vi "HFRR ADV v02.vi"() -> ()   [LabVIEW 2025] (continued)
          tunnel: [FALSE ("RUN") TRUE ("RUN")] -> w2596
          tunnel: [_ 2] -> w2590
          frame False {
          }
          frame True {
          }
        }
        n2286 = case shown="True" w2595 {
          tunnel: [FALSE ("RUN") TRUE ("RUN")] -> w2594
          tunnel: [_ 3] -> w2589
          frame False {
          }
          frame True {
          }
        }
        n2287 = case shown="\"Acquire\"" w2575 {
          tunnel: w2577 -> [_ w2808]
          frame Default {
            w2807 = 0.0 ("output")
            n2288 = local write "PID-out"(w2807) -> ()
            n2289 = local write "Frequency ( Hz )"(w2807) -> ()
          }
          frame "Acquire" {
            n2290 = stacked-sequence {
              frame #0 {
                n2291 = local read "Auto Start Test"() -> (w2810:bool)
                n2292 = case shown="True" w2810 {
                  tunnel: "RUN" -> [w2831 w2834]
                  tunnel: [w2831 w2833] -> w2811
                  frame False {
                  }
                  frame True {
                    n2293 = local read "Auto Start Temp"() -> (w2832:bool)
                    n2294 = Or(x=w2834, y=w2832) -> (x .or. y?=w2833:bool)
                  }
                }
                n2295 = local read "clk"() -> (w2830:dbl)
                n2296 = local read "Save"() -> (w2826:bool)
                n2297 = Equal?(x=w2830, y=0.0) -> (x = y?=w2827:bool)
                n2298 = And(x=w2827, y=w2826) -> (x .and. y?=w2828:bool)
                n2299 = Not(x="Engage") -> (.not. x?=w2817:bool)
                n2300 = case shown="True" w2811 {
                  tunnel: [0.0 w2851] -> w2813
                  frame False {
                    (unwired) TRUE ("Visible")
                    n2301 = local read "Auto Start Test"() -> (w2838:bool)
                    n2302 = local write "Start Time"(TRUE ("Start Time")) -> ()
                    n2303 = property on="Stroke 2" class="DigNum (strict)"("Visible"=FALSE) -> ()  [unwired: 2 in, 2 out]
                    n2304 = case shown="False" w2838 {
                      frame False {
                        n2305 = property on="Heater Button" class="Bool (strict)"("DisabledEnum"=T13."Enabled" ("Disabled")) -> ()  [unwired: 2 in, 2 out]
                        n2306 = property on="Humidity" class="Bool (strict)"("DisabledEnum"=T13."Enabled" ("Disabled")) -> ()  [unwired: 2 in, 2 out]
                      }
                      frame True {
                      }
                    }
                    n2307 = case shown="False" "TestCompFlg" {
                      frame False {
                        n2308 = local read "StartFlg"() -> (w2846:bool)
                        n2309 = case shown="True" w2846 {
                          frame False {
                          }
                          frame True {
                            n2310 = flat-sequence {
                              frame #0 {
                                n2311 = local read "EVENT LOG"() -> (w2848:string)
                                n2312 = call "Event Log.vi"("Content"="Test was interrupted", "EVENT LOG"=w2848) -> ("EVENT LOG"=w2849:string)  [unwired: 8 in, 1 out]
                                n2313 = local write "EVENT LOG"(w2849) -> ()
                              }
                              frame #1 {
                                w2850 = FALSE ("StartFlg")
                                n2314 = local write "Heater Button"(w2850) -> ()
                                n2315 = local write "StartFlg"(w2850) -> ()
                                n2316 = local write "Humidity"(w2850) -> ()
                              }
                            }
                          }
                        }
                      }
                      frame True {
                      }
                    }
                    n2317 = local write "String 14"("Test will autostart once parameters reach the set value." ("String 14")) -> ()
                  }
                  frame True {
                    (unwired) FALSE ("Visible")
                    n2318 = property on="Stroke 2" class="DigNum (strict)"("Visible"=TRUE) -> ()  [unwired: 2 in, 2 out]
                    n2319 = property on="STOP 2" class="Bool (strict)"("Disabled"=u8 2) -> ()  [unwired: 2 in, 2 out]
                    n2320 = local write "String 14"(" Running....." ("String 14")) -> ()
                    n2321 = property on="Heater Button" class="Bool (strict)"("DisabledEnum"=T13."Disabled and Grayed Out" ("Disabled")) -> ()  [unwired: 2 in, 2 out]
                    n2322 = property on="Humidity" class="Bool (strict)"("DisabledEnum"=T13."Disabled and Grayed Out" ("Disabled")) -> ()  [unwired: 2 in, 2 out]
                    n2323 = case shown="True" "Start Time" {
                      selector: "Start Time" -> [_ w2864]
                      frame False {
                      }
                      frame True {
                        n2324 = Not(x=w2864) -> (.not. x?=w2863:bool)
                        n2325 = local write "Start Time"(w2863) -> ()
                        n2326 = local read "EVENT LOG"() -> (w2865:string)
                        n2327 = call "Event Log.vi"("Content"="Test in progress", "EVENT LOG"=w2865) -> ("EVENT LOG"=w2867:string)  [unwired: 8 in, 1 out]
                        n2328 = local write "EVENT LOG"(w2867) -> ()
                      }
                    }
                    n2329 = local read "Set Hz"() -> (w2861:dbl)
                    n2330 = call <vilib>:"Uniform White Noise Waveform.vi"() -> ("signal out"=w2860:waveform(dbl))  [unwired: 10 in, 1 out]
                    n2331 = Add(x=w2861, y=w2860) -> (x+y=w2859:waveform(dbl))
                    n2332 = Multiply(x=w2859, y=ext 0.1) -> (x*y=w2851:waveform(ext))
                    "StartFlg" <- TRUE ("StartFlg")
                  }
                }
                n2333 = case shown="True" w2828 {
                  frame False {
                  }
                  frame True {
                    n2334 = local write "clk"(10.0 ("clk")) -> ()
                    n2335 = Get Date/Time In Seconds() -> (seconds since 1Jan1904=w2870:timestamp)
                    n2336 = To Double Precision Float(number=w2870) -> (double precision float=w2868:dbl)
                    n2337 = local write "acq timer"(w2868) -> ()
                    n2338 = local write "act save time"(w2868) -> ()
                  }
                }
                n2339 = call "Elapsed Time"("Time Target (s)"="Countdown", "Reset"=w2817) -> ("Elapsed Time (s)"=w2822:dbl, "Time has Elapsed"=w2820:bool)  [unwired: 10 in, 6 out]
                "Countdown 2" <- w2822
                n2340 = Subtract(x=w2822, y=2.0) -> (x-y=w2825:dbl)
                n2341 = Less?(x=w2825, y="Countdown") -> (x < y?=w2823:bool)
                n2342 = And(x=w2823, y=w2820) -> (x .and. y?=w2819:bool)
                n2343 = case shown="True" w2819 {
                  frame False {
                  }
                  frame True {
                    (unwired) dbl[] [] ("History Data")
                    n2344 = local write "Engage"(FALSE ("Engage")) -> ()
                    n2345 = local write "RUN"(TRUE ("RUN")) -> ()
                    n2346 = local read "Humidity ( %RH )"() -> (→"Rh Before":dbl)
                  }
                }
                n2347 = local read "Test \nStatus"() -> (w2815:bool)
                n2348 = Select(t=w2813, s=w2815, f=0.0) -> (s? t:f=w2814:dbl)
                n2349 = local write "Frequency ( Hz )"(w2814) -> ()
              }
              frame #1 {
                w2893 = 1000000.0 ("x")
                # "Elapsed time\ncof\nstroke\nAir temp\nTemp\nHumidity"
                # "acq timer\n\nact save time"
                # "convert to microseconds"
                n2350 = local read "COUNT"() -> (w2876:i32)
                n2351 = local read "Rate"() -> (w2889:dbl)
                n2352 = Divide(x=w2893, y=w2889) -> (x/y=w2894:dbl)
                n2353 = Greater Or Equal?(x=w2876, y=250) -> (x >= y?=w2875:bool)
                n2354 = Get Date/Time In Seconds() -> (seconds since 1Jan1904=w2896:timestamp)
                n2355 = case shown="True" w2875 {
                  frame False {
                    n2356 = local read "COUNT"() -> (w2897:i32)
                    n2357 = Increment(x=w2897) -> (x+1=w2898:i32)
                    n2358 = local write "COUNT"(w2898) -> ()
                  }
                  frame True {
                    n2359 = local write "COUNT"(0 ("COUNT")) -> ()
                  }
                }
                n2360 = local read "Samplingtime 2"() -> (w2874:dbl)
                n2361 = local read "act save time"() -> (w2891:dbl)
                n2362 = Divide(x=w2894, y=w2893) -> (x/y=w2892:dbl)
                n2363 = To Double Precision Float(number=w2896) -> (double precision float=w2885:dbl)
                n2364 = Add(x=w2891, y=w2874) -> (x+y=w2890:dbl)
                n2365 = local read "acq timer"() -> (w2895:dbl)
                n2366 = local read "COUNT"() -> (w2878:i32)
                n2367 = Greater Or Equal?(x=w2885, y=w2890) -> (x >= y?=w2873:bool)
                n2368 = Multiply(x=w2892, y=w2878) -> (x*y=w2884:dbl)
                n2369 = Subtract(x=w2885, y=w2895) -> (x-y=w2887:dbl)
                n2370 = local read "Save"() -> (w2888:bool)
                n2371 = Add(x=w2887, y=w2884) -> (x+y=w2871:dbl)
                "Elapsed time 3" <- w2871
                n2372 = And(x=w2873, y=w2888) -> (x .and. y?=w2886:bool)
                n2373 = Divide(x=w2871, y=60.0) -> (x/y=w2882:dbl)
                n2374 = local read "Test \nStatus"() -> (w2872:bool)
                n2375 = local read "clk"() -> (w2879:dbl)
                n2376 = Equal?(x=w2879, y=10.0) -> (x = y?=w2881:bool)
                n2377 = case shown="True" w2886 {
                  tunnel: w2885 -> [_ w2996]
                  tunnel: [FALSE ("Boolean 2") TRUE ("Boolean 2")] -> _
                  frame False {
                  }
                  frame True {
                    w2950 = ";" ("Substring")
                    # "Pid out/\nFreq response value"
                    n2378 = local write "act save time"(w2996) -> ()
                    n2379 = local read "FILE"() -> (w2944:string)
                    n2380 = call "file check.vi"("file name in"=w2944) -> ("error out"=w2947:errorcluster, "file name out"=w2942:string)  [unwired: 9 in]
                    n2381 = call "FILE PATH CREATION.vi"("error in"=w2947, "FILE NAME :"=w2942) -> ("FILE OUT"=w2945:path)  [unwired: 8 in, 1 out]
                    n2382 = Concatenate Strings(w2942, ".dgf" ("Substring")) -> (w2946:string)
                    n2383 = local read "FF 2"() -> (→"Frictional Force ( N )" →"Frictional Force ( N )":dbl)
                    n2384 = Build Path(base path=w2945, name or relative path=w2946) -> (appended path=w2941:path)
                    n2385 = local read "COF 2"() -> (w2955:dbl)
                    "cof" <- w2955
                    "Coefficient of Friction" <- w2955
                    "COF 4" <- w2955
                    "Coefficient of Friction" <- w2955
                    n2386 = local read "TEMP"() -> (w2958:dbl)
                    "Temp" <- w2958
                    "Temperature ( Deg C )" <- w2958
                    n2387 = local read "Humidity ( %RH )"() -> (w2957:dbl)
                    "Humidity ( %RH )" <- w2957
                    "Humidity ( %RH )" <- w2957
                    n2388 = local read "Frequency ( Hz )"() -> (w2964:dbl)
                    n2389 = local read "Elapsed time"() -> (w2989:dbl)
                    n2390 = local read "AIR TEMP"() -> (w2962:dbl)
                    n2391 = local read "PID-out"() -> (w2967:dbl)
                    n2392 = local write "Temperature ( Deg C )"(w2958) -> ()
                    n2393 = Number To Fractional String(number="measured_stroke", width (-)=i16 9 ("precision (6)"), precision (6)=i16 6) -> (F-format string=w2982:string)  [unwired: 1 in]
                    n2394 = Number To Fractional String(number=w2962, width (-)=i16 9 ("precision (6)"), precision (6)=i16 3) -> (F-format string=w2981:string)  [unwired: 1 in]
                    n2395 = Number To Fractional String(number=w2958, width (-)=i16 9 ("precision (6)"), precision (6)=i16 3) -> (F-format string=w2978:string)  [unwired: 1 in]
                    n2396 = Number To Fractional String(number=w2957, width (-)=i16 9 ("precision (6)"), precision (6)=i16 3) -> (F-format string=w2975:string)  [unwired: 1 in]
                    n2397 = Number To Fractional String(number=0.0, width (-)=i16 9 ("precision (6)"), precision (6)=i16 3) -> (F-format string=w2972:string)  [unwired: 1 in]
                    n2398 = Number To Fractional String(number=w2967, width (-)=i16 9 ("precision (6)"), precision (6)=i16 3) -> (F-format string=w2968:string)  [unwired: 1 in]
                    n2399 = Number To Fractional String(number=w2964, width (-)=i16 9 ("precision (6)"), precision (6)=i16 3) -> (F-format string=w2963:string)  [unwired: 1 in]
                    n2400 = Number To Fractional String(number=w2955, width (-)=i16 9 ("precision (6)"), precision (6)=i16 6) -> (F-format string=w2990:string)  [unwired: 1 in]
                    n2401 = Number To Fractional String(number=w2989, width (-)=i16 14 ("precision (6)"), precision (6)=i16 3) -> (F-format string=w2991:string)  [unwired: 1 in]
                    n2402 = Bundle("y"=1.02, "measured_stroke"="measured_stroke", "y"=0.98) -> (w2956:cluster{"y":dbl, "measured_stroke":dbl, "y":dbl})  [unwired: 1 in]
                    n2403 = Number To Fractional String(number="Ambient Humidity :", width (-)=i16 9 ("precision (6)"), precision (6)=i16 6) -> (F-format string=w2948:string)  [unwired: 1 in]
                    n2404 = local read "RUN"() -> (w2954:bool)
                    n2405 = case shown="True" w2954 {
                      tunnel: w2956 -> [_ w3001]
                      tunnel: "measured_stroke" -> [_ w3000]
                      tunnel: "measured_stroke" -> [_ w2999]
                      tunnel: "measured_stroke" -> [_ w2998]
                      frame False {
                      }
                      frame True {
                        "Stroke ( mm )" <- w3001
                        "Stroke ( mm )" <- w3001
                        "Stroke 4" <- w3000
                        "Stroke 3" <- w2999
                        "Stroke 2" <- w2998
                      }
                    }
                    n2406 = Concatenate Strings(w2991, w2950, w2990, w2950, w2982, w2950, w2981, w2950, w2978, w2950, w2975, w2950, w2972, w2950, w2968, w2950, w2963, w2950, w2948, "\r") -> (w2988:string)
                    n2407 = call <vilib>:"Write Characters To File.vi"("append to file? (new file:F)"=TRUE, "character string"=w2988, "file path (dialog if empty)"=w2941) -> ()  [unwired: 2 in, 1 out]
                    "refresh flag" <- TRUE ("refresh flag")
                  }
                }
                n2408 = case shown="True" w2872 {
                  tunnel: w2882 -> [_ w2908]
                  tunnel: w2887 -> [_ w2918]
                  tunnel: [0.0 w2914] -> _
                  tunnel: w2881 -> [_ w2913]
                  tunnel: [0.0 w2912] -> _
                  tunnel: w2871 -> [_ w2912]
                  tunnel: w2885 -> [w2901 _]
                  frame False {
                    n2409 = local write "acq timer"(w2901) -> ()
                    n2410 = local write "Test Duration Status"(0.0 ("Test Duration Status")) -> ()
                  }
                  frame True {
                    n2411 = local read "Set Hz"() -> (w2915:dbl)
                    n2412 = local write "Elapsed time"(w2908) -> ()
                    n2413 = local read "test time"() -> (w2907:dbl)
                    n2414 = Multiply(x=w2918, y=w2915) -> (x*y=w2917:dbl)
                    n2415 = case shown="False" w2913 {
                      tunnel: w2917 -> [w2919 _]
                      tunnel: [w2919 1.0] -> w2914
                      frame False {
                        n2416 = local write "Cycles elapsed"(w2919) -> ()
                      }
                      frame True {
                      }
                    }
                    n2417 = Greater?(x=w2908, y=w2907) -> (0:w2916:bool)
                    n2418 = Subtract(x=w2907, y=w2908) -> (x-y=w2906:dbl)
                    "time" <- w2906
                    n2419 = Multiply(x=w2906, y=60.0) -> (x*y=w2905:dbl)
                    n2420 = local write "Time Remaining"(w2905) -> ()
                    n2421 = local write "Remaining Time"(w2905) -> ()
                    n2422 = case shown="True" w2916 {
                      frame False {
                      }
                      frame True {
                        w2923 = T13."Enabled" ("Disabled")
                        w2921 = FALSE ("TEST FILE NAM,E SAVED")
                        w2926 = "" ("FILE")
                        w2927 = TRUE ("Visible")
                        n2423 = local write "Humidity"(FALSE ("Humidity")) -> ()
                        n2424 = local write "RUN"(FALSE ("OK Button 2")) -> ()
                        n2425 = local write "Heater Button"(FALSE ("Heater Button")) -> ()
                        n2426 = local write "Auto Start Test"(FALSE ("Auto Start Test")) -> ()
                        n2427 = local write "TestCompFlg"(TRUE ("StpFlg")) -> ()
                        n2428 = local read "Humidity ( %RH )"() -> (→"Rh After":dbl)
                        n2429 = property on="STOP 2" class="Bool (strict)"("Disabled"=u8 0) -> ()  [unwired: 2 in, 2 out]
                        n2430 = local read "EVENT LOG"() -> (w2932:string)
                        n2431 = call "Event Log.vi"("Content"="Test Completed", "EVENT LOG"=w2932) -> ("EVENT LOG"=w2931:string)  [unwired: 8 in, 1 out]
                        n2432 = property on="RUN" class="Bool (strict)"("Visible"=w2927) -> ()  [unwired: 2 in, 2 out]
                        n2433 = property on="Auto Start Test" class="Bool (strict)"("Visible"=w2927) -> ()  [unwired: 2 in, 2 out]
                        n2434 = local write "Batch Ref Num :"(w2926) -> ()
                        n2435 = local write "FILE"(w2926) -> ()
                        n2436 = local write "EVENT LOG"(w2931) -> ()
                        n2437 = local write "TEST FILE NAM,E SAVED"(w2921) -> ()
                        n2438 = local write "Fuel Discription :"(w2926) -> ()
                        n2439 = local write "START TEMP"(w2921) -> ()
                        n2440 = local write "Remarks :"(w2926) -> ()
                        n2441 = local write "Main Dashboard Buttons"(T1."Imaging" ("Main Dashboard Buttons")) -> ()
                        n2442 = local write "Main Tab"(T2."Adv Scar" ("Main Tab")) -> ()
                        n2443 = local write "Command"("0") -> ()
                        n2444 = property on="FRICVALZ 2" class="Bool (strict)"("DisabledEnum"=w2923) -> ()  [unwired: 2 in, 2 out]
                        n2445 = property on="FRICVALZ 3" class="Bool (strict)"("DisabledEnum"=w2923) -> ()  [unwired: 2 in, 2 out]
                        n2446 = property on="FRICVALZ 4" class="Bool (strict)"("DisabledEnum"=w2923) -> ()  [unwired: 2 in, 2 out]
                      }
                    }
                    n2447 = Divide(x=w2908, y=w2907) -> (x/y=w2911:dbl)
                    n2448 = Multiply(x=w2911, y=100.0) -> (x*y=w2909:dbl)
                    n2449 = local write "Test Duration Status"(w2909) -> ()
                  }
                }
              }
              frame #2 {
                n2450 = case shown="True" "Heater Button" {
                  tunnel: [0.0 ("output") w3024] -> w3002
                  frame False {
                    w3005 = TRUE ("tmpchk")
                    n2451 = local read "TEMP"() -> (w3006:dbl)
                    n2452 = local write "Temp ini"(w3006) -> ()
                    n2453 = local write "Reset 4"(w3005) -> ()
                    n2454 = local write "tmpchk"(w3005) -> ()
                    n2455 = local write "reinit"(TRUE ("reinit")) -> ()
                    n2456 = local write "manual temp log"(TRUE ("manual temp log")) -> ()
                  }
                  frame True {
                    # "Logic to turn off\nthe heater when \ntemp is not rising.\nTime - 60 sec\nDelta t- 5°c"
                    n2457 = local read "Temp ini"() -> (w3013:dbl)
                    n2458 = local read "Auto Start Test"() -> (w3009:bool)
                    n2459 = Less?(x=w3013, y=53.0) -> (x < y?=w3011:bool)
                    n2460 = case shown="False" w3009 {
                      frame False {
                        n2461 = local read "Set Temp"() -> (w3033:dbl)
                        n2462 = local read "TEMP"() -> (w3032:dbl)
                        n2463 = Subtract(x=w3033, y=w3032) -> (x-y=w3031:dbl)
                        n2464 = Absolute Value(x=w3031) -> (abs(x)=w3030:dbl)
                        n2465 = Less?(x=w3030, y=0.5) -> (x < y?=w3028:bool)
                        n2466 = case shown="True" w3028 {
                          tunnel: "manual temp log" -> [_ w3034]
                          frame False {
                          }
                          frame True {
                            n2467 = case shown="True" w3034 {
                              selector: w3034 -> [_ w3035]
                              frame False {
                              }
                              frame True {
                                # "#Event log"
                                n2468 = Not(x=w3035) -> (.not. x?=w3036:bool)
                                n2469 = local write "manual temp log"(w3036) -> ()
                                n2470 = local read "EVENT LOG"() -> (w3039:string)
                                n2471 = call "Event Log.vi"("Content"="Target Temperature reached", "EVENT LOG"=w3039) -> ("EVENT LOG"=w3038:string)  [unwired: 8 in, 1 out]
                                n2472 = local write "EVENT LOG"(w3038) -> ()
                              }
                            }
                          }
                        }
                      }
                      frame True {
                        n2473 = local write "manual temp log"(TRUE ("manual temp log")) -> ()
                      }
                    }
                    n2474 = And(x="tmpchk", y=w3011) -> (x .and. y?=w3014:bool)
                    n2475 = case shown="True" w3014 {
                      frame False {
                      }
                      frame True {
                        n2476 = call "Elapsed Time8"("Time Target (s)"=300.0, "Reset"="Reset 4") -> ("Time has Elapsed"=w3041:bool)  [unwired: 10 in, 7 out]
                        n2477 = flat-sequence {
                          tunnel: w3041 -> [_]
                          frame #0 {
                            n2478 = local write "Reset 4"(FALSE ("Reset 4")) -> ()
                          }
                        }
                        n2479 = case shown="True" w3041 {
                          frame False {
                          }
                          frame True {
                            n2480 = local read "Temp ini"() -> (w3048:dbl)
                            n2481 = Add(x=w3048, y=5.0) -> (x+y=w3046:dbl)
                            n2482 = local read "TEMP"() -> (w3049:dbl)
                            n2483 = Greater?(x=w3049, y=w3046) -> (0:w3047:bool)
                            n2484 = case shown="False" w3047 {
                              frame False {
                                n2485 = local write "Heater Button"(FALSE ("Heater Button")) -> ()
                              }
                              frame True {
                                n2486 = local write "tmpchk"(FALSE ("tmpchk")) -> ()
                              }
                            }
                          }
                        }
                      }
                    }
                    n2487 = local read "Set Temp"() -> (w3022:dbl)
                    n2488 = local read "TEMP"() -> (w3016:dbl)
                    n2489 = call-poly <vilib>:"PID.vi"("reinitialize? (F)"="reinit", "dt (s)"=-1.0, "process variable"=w3016, "setpoint"=w3022) -> ("output"=w3019:dbl)  [unwired: 6 in, 1 out]
                    n2490 = Subtract(x=w3022, y=w3016) -> (x-y=w3023:dbl)
                    n2491 = Add(x=w3022, y=0.5) -> (x+y=w3020:dbl)
                    n2492 = Greater Or Equal?(x=w3016, y=w3020) -> ()  [unwired: 1 out]
                    n2493 = Select(t=0.0, s=FALSE, f=w3019) -> (s? t:f=w3018:dbl)
                    "PID output" <- w3018
                    n2494 = flat-sequence {
                      tunnel: w3018 -> [w3052]
                      tunnel: [w3052] -> w3024
                      frame #0 {
                        n2495 = local write "reinit"(FALSE ("reinit")) -> ()
                      }
                    }
                    n2496 = Bundle(w3023, "output"=w3018, "TEMP"=w3016) -> ()  [unwired: 1 in, 1 out]
                  }
                }
                "PID-out" <- w3002
              }
              frame #3 {
                n2497 = local read "TEMP"() -> (w3054:dbl)
                n2498 = Greater Or Equal?(x=w3054, y="Set Temp 2") -> (x >= y?=w3059:bool)
                n2499 = case shown="True" w3059 {
                  tunnel: [FALSE TRUE] -> w3057
                  frame False {
                  }
                  frame True {
                  }
                }
                "Status 13" <- w3057
                n2500 = And(x=w3057, y="trip1 8") -> (x .and. y?=w3056:bool)
                n2501 = case shown="True" w3056 {
                  frame False {
                    n2502 = local write "Heater Trip Temp"(TRUE ("Heater Trip Temp")) -> ()
                  }
                  frame True {
                    w3062 = FALSE ("OK Button 2")
                    n2503 = case shown="True" "Heater Trip Temp" {
                      selector: "Heater Trip Temp" -> [_ w3064]
                      frame False {
                      }
                      frame True {
                        n2504 = Not(x=w3064) -> (.not. x?=w3063:bool)
                        n2505 = local read "EVENT LOG"() -> (w3067:string)
                        n2506 = local write "Heater Trip Temp"(w3063) -> ()
                        n2507 = call "Event Log.vi"("Content"="Heater Trip", "EVENT LOG"=w3067) -> ("EVENT LOG"=w3066:string)  [unwired: 8 in, 1 out]
                        n2508 = local write "EVENT LOG"(w3066) -> ()
                      }
                    }
                    n2509 = local write "RUN"(w3062) -> ()
                    n2510 = property on="Auto Start Test" class="Bool (strict)"("Value"=w3062) -> ()  [unwired: 2 in, 2 out]
                    n2511 = local write "Heater Button"(w3062) -> ()
                  }
                }
              }
            }
            n2512 = case shown="False" w2808 {
              frame False {
                n2513 = disable-structure shown="Enabled" {
                  frame Disabled {
                    n2514 = stacked-sequence {
                      frame #0 {
                        n2515 = local write "RUN"(FALSE ("OK Button 2")) -> ()
                      }
                      frame #1 {
                      }
                    }
                  }
                  frame Enabled {
                  }
                }
              }
              frame True {
              }
            }
          }
        }
        n2516 = local read "airtempflg"() -> (w2600:bool)
        n2517 = Or(x=w2600, y=w2598) -> (x .or. y?=w2601:bool)
        n2518 = Insert Into Array(array=string[] ["Air Temperature has reached set value,", "Humidity has reached set value,", "Sample Temperaturehas reached set value,", ""], index=0, new element="") -> (w2586:string[])
        n2519 = Build Array(w2591, w2590, w2589) -> (w2587:i32[])
        n2520 = disable-structure shown="Disabled" {
          disable-tunnel: w2601 -> [w2678 _]
          disable-tunnel: w2596 -> [w2677 _]
          disable-tunnel: w2594 -> [w2676 _]
          frame Disabled {
            n2521 = Compound Arithmetic op=AND(w2678, w2677, w2676) -> ()  [unwired: 1 out]
            n2522 = case shown="True" {
              selector: _ -> [_ _]
              frame False {
              }
              frame True {
                w2679 = FALSE ("autostrtflg")
                n2523 = local write "RUN"(TRUE ("RUN")) -> ()
                n2524 = local write "autostrtflg"(w2679) -> ()
                n2525 = local write "autostart"(w2679) -> ()
                n2526 = local write "String 14"(" Running....." ("String 14")) -> ()
              }
            }
          }
          frame Enabled {
          }
        }
        n2527 = for {
          tunnel: w2587 -> [w2729] mode=indexing
          tunnel: w2586 -> [w2728]
          shift-right: [w2725] -> w2585
          shift-left: "" -> [w2727]
          n2528 = Index Array(array=w2728, index=w2729) -> (element=w2726:string)
          n2529 = Concatenate Strings(w2726, w2727) -> (w2725:string)
        }
        n2530 = local write "autostart 2"(w2585) -> ()
        n2531 = local read "Reset Graph"() -> (w2574:bool)
        n2532 = case shown="True" w2574 {
          selector: w2574 -> [_ w2628]
          frame False {
          }
          frame True {
            w2642 = 0.0 ("X Scale.Range:Maximum")
            n2533 = Not(x=w2628) -> (.not. x?=w2627:bool)
            n2534 = local write "Reset Graph"(w2627) -> ()
            n2535 = property on="Electrical Contact Resistance ( % )" class="WFChart (strict)"("XScale.Maximum"=600.0 ("X Scale.Range:Maximum"), "XScale.Minimum"=0.0 ("X Scale.Range:Minimum"), "YScale.Maximum"=100.0 ("Y Scale.Range:Maximum"), "YScale.Minimum"=0.0 ("Y Scale.Range:Minimum")) -> ()  [unwired: 2 in, 2 out]
            n2536 = property on="Frictional Force ( N )" class="WFChart (strict)"("XScale.Maximum"=600.0 ("X Scale.Range:Maximum"), "XScale.Minimum"=0.0 ("X Scale.Range:Minimum"), "YScale.Maximum"=100.0 ("Y Scale.Range:Maximum"), "YScale.Minimum"=0.0 ("Y Scale.Range:Minimum")) -> ()  [unwired: 2 in, 2 out]
            n2537 = property on="Temperature ( Deg C )" class="WFChart (strict)"("XScale.Maximum"=600.0 ("X Scale.Range:Maximum"), "XScale.Minimum"=0.0 ("X Scale.Range:Minimum"), "YScale.Maximum"=100.0 ("Y Scale.Range:Maximum"), "YScale.Minimum"=0.0 ("Y Scale.Range:Minimum")) -> ()  [unwired: 2 in, 2 out]
            n2538 = property on="Humidity ( %RH )" class="WFChart (strict)"("XScale.Maximum"=600.0 ("X Scale.Range:Maximum"), "XScale.Minimum"=0.0 ("X Scale.Range:Minimum"), "YScale.Maximum"=100.0 ("Y Scale.Range:Maximum"), "YScale.Minimum"=0.0 ("Y Scale.Range:Minimum")) -> ()  [unwired: 2 in, 2 out]
            n2539 = property on="Stroke ( mm )" class="WFChart (strict)"("XScale.Maximum"=600.0 ("X Scale.Range:Maximum"), "XScale.Minimum"=0.0 ("X Scale.Range:Minimum"), "YScale.Maximum"=100.0 ("Y Scale.Range:Maximum"), "YScale.Minimum"=0.0 ("Y Scale.Range:Minimum")) -> ()  [unwired: 2 in, 2 out]
            n2540 = property on="Coefficient of Friction" class="WFChart (strict)"("XScale.Maximum"=600.0 ("X Scale.Range:Maximum"), "XScale.Minimum"=0.0 ("X Scale.Range:Minimum"), "YScale.Maximum"=100.0 ("Y Scale.Range:Maximum"), "YScale.Minimum"=0.0 ("Y Scale.Range:Minimum")) -> ()  [unwired: 2 in, 2 out]
            n2541 = property on="Electrical Contact Resistance ( % )" class="WFChart (strict)"("XScale.Minimum"=0.0 ("X Scale.Range:Minimum"), "XScale.Maximum"=600.0 ("X Scale.Range:Maximum"), "YScale.Minimum"=0.0 ("Y Scale.Range:Minimum"), "YScale.Maximum"=100.0 ("Y Scale.Range:Maximum")) -> ()  [unwired: 2 in, 2 out]
            n2542 = property on="Temperature ( Deg C )" class="WFChart (strict)"("XScale.Minimum"=0.0 ("X Scale.Range:Minimum"), "XScale.Maximum"=600.0 ("X Scale.Range:Maximum"), "YScale.Minimum"=0.0 ("Y Scale.Range:Minimum"), "YScale.Maximum"=100.0 ("Y Scale.Range:Maximum")) -> ()  [unwired: 2 in, 2 out]
            n2543 = property on="Coefficient of Friction" class="WFChart (strict)"("XScale.Minimum"=0.0 ("X Scale.Range:Minimum"), "XScale.Maximum"=600.0 ("X Scale.Range:Maximum"), "YScale.Maximum"=1.0 ("X Scale.Range:Minimum"), "YScale.Minimum"=0.0 ("X Scale.Range:Minimum")) -> ()  [unwired: 2 in, 2 out]
            n2544 = property on="Frictional Force ( N )" class="WFChart (strict)"("XScale.Maximum"=600.0 ("X Scale.Range:Maximum"), "XScale.Minimum"=w2642, "YScale.Maximum"=10.0 ("Y Scale.Range:Maximum"), "YScale.Minimum"=w2642) -> ()  [unwired: 2 in, 2 out]
            n2545 = property on="Stroke ( mm )" class="WFChart (strict)"("XScale.Maximum"=600.0 ("X Scale.Range:Maximum"), "XScale.Minimum"=0.0 ("X Scale.Range:Minimum"), "YScale.Maximum"=100.0 ("Y Scale.Range:Maximum"), "YScale.Minimum"=0.0 ("Y Scale.Range:Minimum")) -> ()  [unwired: 2 in, 2 out]
            n2546 = property on="Humidity ( %RH )" class="WFChart (strict)"("XScale.Maximum"=600.0 ("X Scale.Range:Maximum"), "XScale.Minimum"=0.0 ("X Scale.Range:Minimum"), "YScale.Maximum"=100.0 ("Y Scale.Range:Maximum"), "YScale.Minimum"=0.0 ("Y Scale.Range:Minimum")) -> ()  [unwired: 2 in, 2 out]
          }
        }
      }
      frame "Compare Files" {
        # "Elapsed time\ncof\nstroke\nAir temp\nTemp\nHumidity"
        n2547 = case shown="True" "RSTV1 2" {
          frame False {
          }
          frame True {
            n2548 = property on="Humidity ( %RH )" class="XYGraph (strict)"("Y Scale.Display Format:Precision"=u8 0 ("Y Scale.Format & Precision:Precision")) -> ()  [unwired: 2 in, 2 out]
            n2549 = property on="Humidity ( %RH )" class="XYGraph (strict)"("X Scale.Range:Minimum"=0.0, "X Scale.Range:Maximum"=75.0, "Y Scale.Range:Minimum"=48.0, "Y Scale.Range:Maximum"=58.0) -> ()  [unwired: 2 in, 2 out]
          }
        }
        n2550 = case shown="True" "RST CP 2" {
          frame False {
          }
          frame True {
            n2551 = property on="XY Graph 13" class="XYGraph (strict)"("Y Scale.Display Format:Precision"=u8 0 ("Y Scale.Format & Precision:Precision")) -> ()  [unwired: 2 in, 2 out]
            n2552 = property on="XY Graph 13" class="XYGraph (strict)"("X Scale.Range:Minimum"=0.0, "X Scale.Range:Maximum"=75.0, "Y Scale.Range:Minimum"=0.0, "Y Scale.Range:Maximum"=100.0) -> ()  [unwired: 2 in, 2 out]
          }
        }
        n2553 = case shown="True" "RST CP" {
          frame False {
          }
          frame True {
            n2554 = property on="Sample Temperature ( °C )" class="XYGraph (strict)"("Y Scale.Display Format:Precision"=u8 2 ("Y Scale.Format & Precision:Precision")) -> ()  [unwired: 2 in, 2 out]
            n2555 = property on="Sample Temperature ( °C )" class="XYGraph (strict)"("X Scale.Range:Minimum"=0.0, "X Scale.Range:Maximum"=75.0, "Y Scale.Range:Minimum"=58.0, "Y Scale.Range:Maximum"=62.0) -> ()  [unwired: 2 in, 2 out]
          }
        }
        n2556 = case shown="True" "RSTV1 3" {
          frame False {
          }
          frame True {
            n2557 = property on="Air Temperature  ( °C )" class="XYGraph (strict)"("Y Scale.Display Format:Precision"=u8 2 ("Y Scale.Format & Precision:Precision")) -> ()  [unwired: 2 in, 2 out]
            n2558 = property on="Air Temperature  ( °C )" class="XYGraph (strict)"("X Scale.Range:Minimum"=0.0 ("Y Scale.Range:Minimum"), "X Scale.Range:Maximum"=75.0 ("Y Scale.Range:Maximum"), "Y Scale.Range:Minimum"=20.0 ("X Scale.Range:Minimum"), "Y Scale.Range:Maximum"=26.0 ("X Scale.Range:Maximum")) -> ()  [unwired: 2 in, 2 out]
          }
        }
        n2559 = case shown="True" "RSTV1 4" {
          frame False {
          }
          frame True {
            n2560 = property on="Stroke ( mm )" class="XYGraph (strict)"("Y Scale.Display Format:Precision"=u8 2 ("Y Scale.Format & Precision:Precision")) -> ()  [unwired: 2 in, 2 out]
            n2561 = property on="Stroke ( mm )" class="XYGraph (strict)"("X Scale.Range:Minimum"=0.0 ("Y Scale.Range:Maximum"), "X Scale.Range:Maximum"=75.0 ("X Scale.Range:Minimum"), "Y Scale.Range:Minimum"=0.98, "Y Scale.Range:Maximum"=1.02) -> ()  [unwired: 2 in, 2 out]
          }
        }
        n2562 = case shown="True" "rstv2" {
          frame False {
          }
          frame True {
            n2563 = property on="Coefficient Of Friction" class="XYGraph (strict)"("Y Scale.Display Format:Precision"=u8 3 ("Y Scale.Format & Precision:Precision")) -> ()  [unwired: 2 in, 2 out]
            n2564 = property on="Coefficient Of Friction" class="XYGraph (strict)"("X Scale.Range:Minimum"=0.0 ("Y Scale.Range:Maximum"), "X Scale.Range:Maximum"=75.0, "Y Scale.Range:Minimum"=0.0, "Y Scale.Range:Maximum"=1.0 ("X Scale.Range:Minimum")) -> ()  [unwired: 2 in, 2 out]
          }
        }
        n2565 = case shown="True" "RST CP 3" {
          frame False {
          }
          frame True {
            n2566 = property on="Air Temp ( °C ) vs Humidity ( % RH )" class="XYGraph (strict)"("X Scale.Range:Minimum"=18.0, "X Scale.Range:Maximum"=28.0 ("X Scale.Range:Minimum"), "Y Scale.Range:Minimum"=30.0 ("X Scale.Range:Minimum"), "Y Scale.Range:Maximum"=70.0 ("X Scale.Range:Minimum")) -> ()  [unwired: 2 in, 2 out]
          }
        }
        n2567 = case shown="True" "OPEN 1" {
          frame False {
          }
          frame True {
            (unwired) 0  # existing file
            w3343 = "Choose a datalog file to open"  # prompt
            n2568 = local write "OPEN 1"(FALSE ("OPEN 1")) -> ()
            n2569 = String To Path(string="C:\\LAB-IQ\\Data\\") -> (path=w3328:path)
            n2570 = File Dialog(6:"*.dgf" ("pattern"), 7:w3343, 11:w3328) -> (0:w3326:errorcluster, 3:w3334:path)  [unwired: 4 in, 2 out]
            n2571 = Unbundle(w3326) -> ()  [unwired: 3 out]
            n2572 = Strip Path(path=w3334) -> (name=w3333:string)  [unwired: 1 out]
            n2573 = Path To String(path=w3334) -> (string=w3329:string)
            "string1" <- w3329
            n2574 = Match Pattern(string=w3333, regular expression=".dgf") -> (before substring=→"String Control":string)  [unwired: 1 in, 3 out]
            n2575 = Match Pattern(string=w3329, regular expression=".dgf" ("substring (\"\")")) -> (before substring=w3339:string)  [unwired: 1 in, 3 out]
            n2576 = Concatenate Strings(w3339, ".duf" ("Substring")) -> (w3335:string)
            n2577 = String To Path(string=w3335) -> (path=w3340:path)
            n2578 = call <vilib>:"Read Characters From File.vi"("file path (dialog if empty)"=w3340, "start of read offset (chars.:0)"=60 ("start of read offset (chars.: 0)")) -> ("character string"=→"String Control 2":string)  [unwired: 4 in, 3 out]
          }
        }
        n2579 = case shown="True" "OPEN 2" {
          frame False {
          }
          frame True {
            (unwired) 0  # existing file
            w3361 = "Choose a datalog file to open"  # prompt
            n2580 = local write "OPEN 2"(FALSE ("OPEN 1")) -> ()
            n2581 = String To Path(string="C:\\LAB-IQ\\Data\\") -> (path=w3346:path)
            n2582 = File Dialog(6:"*.dgf" ("pattern"), 7:w3361, 11:w3346) -> (0:w3344:errorcluster, 3:w3352:path)  [unwired: 4 in, 2 out]
            n2583 = Unbundle(w3344) -> ()  [unwired: 3 out]
            n2584 = Strip Path(path=w3352) -> (name=w3350:string)  [unwired: 1 out]
            n2585 = Path To String(path=w3352) -> (string=w3347:string)
            "string1 2" <- w3347
            n2586 = Match Pattern(string=w3350, regular expression=".dgf") -> (before substring=→"String Control 3":string)  [unwired: 1 in, 3 out]
            n2587 = Match Pattern(string=w3347, regular expression=".dgf" ("substring (\"\")")) -> (before substring=w3358:string)  [unwired: 1 in, 3 out]
            n2588 = Concatenate Strings(w3358, ".duf" ("Substring")) -> (w3355:string)
            n2589 = String To Path(string=w3355) -> (path=w3353:path)
            n2590 = call <vilib>:"Read Characters From File.vi"("file path (dialog if empty)"=w3353, "start of read offset (chars.:0)"=60 ("start of read offset (chars.: 0)")) -> ("character string"=→"String Control 4":string)  [unwired: 4 in, 3 out]
          }
        }
        n2591 = case shown="True" "OPEN 3" {
          frame False {
          }
          frame True {
            (unwired) 0  # existing file
            w3379 = "Choose a datalog file to open"  # prompt
            n2592 = local write "OPEN 3"(FALSE ("OPEN 1")) -> ()
            n2593 = String To Path(string="C:\\LAB-IQ\\Data\\") -> (path=w3364:path)
            n2594 = File Dialog(6:"*.dgf" ("pattern"), 7:w3379, 11:w3364) -> (0:w3362:errorcluster, 3:w3370:path)  [unwired: 4 in, 2 out]
            n2595 = Unbundle(w3362) -> ()  [unwired: 3 out]
            n2596 = Strip Path(path=w3370) -> (name=w3368:string)  [unwired: 1 out]
            n2597 = Path To String(path=w3370) -> (string=w3365:string)
            "string1 3" <- w3365
            n2598 = Match Pattern(string=w3368, regular expression=".dgf") -> (before substring=→"String Control 5":string)  [unwired: 1 in, 3 out]
            n2599 = Match Pattern(string=w3365, regular expression=".dgf" ("substring (\"\")")) -> (before substring=w3375:string)  [unwired: 1 in, 3 out]
            n2600 = Concatenate Strings(w3375, ".duf" ("Substring")) -> (w3372:string)
            n2601 = String To Path(string=w3372) -> (path=w3376:path)
            n2602 = call <vilib>:"Read Characters From File.vi"("file path (dialog if empty)"=w3376, "start of read offset (chars.:0)"=60 ("start of read offset (chars.: 0)")) -> ("character string"=→"String Control 6":string)  [unwired: 4 in, 3 out]
          }
        }
        n2603 = case shown="True" "OPEN 4" {
          frame False {
          }
          frame True {
            (unwired) 0  # existing file
            w3397 = "Choose a datalog file to open"  # prompt
            n2604 = local write "OPEN 4"(FALSE ("OPEN 1")) -> ()
            n2605 = String To Path(string="C:\\LAB-IQ\\Data\\") -> (path=w3382:path)
            n2606 = File Dialog(6:"*.dgf" ("pattern"), 7:w3397, 11:w3382) -> (0:w3380:errorcluster, 3:w3388:path)  [unwired: 4 in, 2 out]
            n2607 = Unbundle(w3380) -> ()  [unwired: 3 out]
            n2608 = Strip Path(path=w3388) -> (name=w3386:string)  [unwired: 1 out]
            n2609 = Path To String(path=w3388) -> (string=w3383:string)
            "string1 4" <- w3383
            n2610 = Match Pattern(string=w3386, regular expression=".dgf") -> (before substring=→"String Control 7":string)  [unwired: 1 in, 3 out]
            n2611 = Match Pattern(string=w3383, regular expression=".dgf" ("substring (\"\")")) -> (before substring=w3393:string)  [unwired: 1 in, 3 out]
            n2612 = Concatenate Strings(w3393, ".duf" ("Substring")) -> (w3390:string)
            n2613 = String To Path(string=w3390) -> (path=w3394:path)
            n2614 = call <vilib>:"Read Characters From File.vi"("file path (dialog if empty)"=w3394, "start of read offset (chars.:0)"=60 ("start of read offset (chars.: 0)")) -> ("character string"=→"String Control 8":string)  [unwired: 4 in, 3 out]
          }
        }
      }
      frame "About" {
        # "Elapsed time\ncof\nstroke\nmean pos\nTemp\nHumidity"
        n2615 = disable-structure shown="Disabled" {
          frame Disabled {
            n2616 = case shown="True" "Export" {
              frame False {
              }
              frame True {
                w3419 = "                                      " ("string")
                w3421 = "\r"
                (unwired) i16 6 ("width (-)")
                w3498 = "\r"
                w3430 = "\r"
                n2617 = local write "Export"(FALSE ("Export")) -> ()
                n2618 = local read "String 29"() -> (w3467:string)
                n2619 = local read "String 34"() -> (w3455:string)
                n2620 = local read "String 35"() -> (w3450:string)
                n2621 = local read "String 37"() -> (w3446:string)
                n2622 = local read "String 36"() -> (w3443:string)
                n2623 = local read "String 38"() -> (w3440:string)
                n2624 = local read "String 39"() -> (w3437:string)
                n2625 = Match Pattern(string=w3467, regular expression=".dwm") -> (before substring=w3463:string)  [unwired: 1 in, 3 out]
                "before substring" <- w3463
                n2626 = local read "S 38"() -> (w3458:string)
                n2627 = local read "S 39"() -> (w3451:string)
                n2628 = local read "Temperature before test 2"() -> (w3487:dbl)
                n2629 = local read "Temperature after test 2"() -> (w3492:dbl)
                n2630 = local read "Humidity before test 2"() -> (w3473:dbl)
                n2631 = local read "Humidity after test 2"() -> (w3488:dbl)
                n2632 = local read "MWSD 2"() -> (w3484:dbl)
                n2633 = local read "WS1.4 2"() -> (w3500:dbl)
                n2634 = local read "HCF 2"() -> (w3496:dbl)
                n2635 = local read "AVP 2"() -> (w3485:dbl)
                n2636 = Concatenate Strings("1," ("string"), w3458) -> (w3457:string)
                n2637 = Concatenate Strings("2," ("string"), w3455) -> (w3454:string)
                n2638 = Concatenate Strings("3," ("string"), w3451) -> (w3453:string)
                n2639 = Concatenate Strings("4," ("string"), w3450) -> (w3449:string)
                n2640 = Concatenate Strings("5," ("string"), w3446) -> (w3447:string)
                n2641 = Concatenate Strings("6," ("string"), w3443) -> (w3444:string)
                n2642 = Concatenate Strings("7," ("string"), w3440) -> (w3441:string)
                n2643 = Concatenate Strings("8," ("string"), w3437) -> (w3438:string)
                n2644 = local read "Sample ID"() -> (w3505:string)
                n2645 = case shown="\"xlx\"" "Select File Type" {
                  tunnel: w3463 -> [w3508 w3510 w3512]
                  tunnel: [w3506 w3511 w3513] -> w3462
                  frame "xlx" {
                    n2646 = Concatenate Strings(w3508, ".xls" ("string")) -> (w3506:string)
                  }
                  frame "csv" {
                    n2647 = Concatenate Strings(w3510, ".csv" ("string")) -> (w3511:string)
                  }
                  frame "txt" {
                    n2648 = Concatenate Strings(w3512, ".txt" ("string")) -> (w3513:string)
                  }
                }
                n2649 = local read "Test Date"() -> (w3504:string)
                n2650 = local read "String 45"() -> (w3418:string)
                n2651 = local read "String 31"() -> (w3503:string)
                n2652 = local read "String 32"() -> (w3502:string)
                n2653 = local read "TITTLE"() -> (w3426:string)
                n2654 = Number To Fractional String(number=w3473, width (-)=i16 6, precision (6)=i16 2) -> (F-format string=w3472:string)  [unwired: 1 in]
                n2655 = Number To Fractional String(number=w3487, width (-)=i16 6, precision (6)=i16 2) -> (F-format string=w3493:string)  [unwired: 1 in]
                n2656 = Number To Fractional String(number=w3488, width (-)=i16 6, precision (6)=i16 2) -> (F-format string=w3486:string)  [unwired: 1 in]
                n2657 = Number To Fractional String(number=w3492, width (-)=i16 6, precision (6)=i16 2) -> (F-format string=w3491:string)  [unwired: 1 in]
                n2658 = Number To Fractional String(number=w3484, width (-)=i16 6, precision (6)=i16 2) -> (F-format string=w3482:string)  [unwired: 1 in]
                n2659 = Number To Fractional String(number=w3485, width (-)=i16 6, precision (6)=i16 2) -> (F-format string=w3483:string)  [unwired: 1 in]
                n2660 = Number To Fractional String(number=w3496, width (-)=i16 6, precision (6)=i16 2) -> (F-format string=w3497:string)  [unwired: 1 in]
                n2661 = Number To Fractional String(number=w3500, precision (6)=i16 2) -> (F-format string=w3501:string)  [unwired: 2 in]
                n2662 = local read "s.NO"() -> (w3420:string)
                n2663 = Concatenate Strings("=" ("string"), w3426) -> (w3425:string)
                n2664 = Concatenate Strings("S.No," ("string"), "                                       Parameters" ("string")) -> (w3431:string)
                n2665 = Concatenate Strings(w3498, w3457, w3472, w3498, w3454, w3493, w3498, w3453, w3486, w3498, w3449, w3491, w3498, w3447, w3482, w3498, w3444, w3483, w3498, w3441, w3497, w3498, w3438, w3501) -> (w3460:string)
                n2666 = Concatenate Strings(w3430, "," ("string"), w3418, w3420, w3419, w3502, w3505, w3419, w3503, w3504, w3430) -> (w3428:string)
                n2667 = local read "Tested by"() -> (w3434:string)
                n2668 = local read "String 33"() -> (w3435:string)
                n2669 = Concatenate Strings("," ("string"), "                                                                             " ("string")) -> (w3423:string)
                n2670 = Concatenate Strings(w3425, w3421, w3428, w3421, w3431, w3460, w3421, w3423, w3435, w3434) -> (→"export":string)
                n2671 = String To Path(string=w3462) -> (path=w3469:path)
                n2672 = local read "export"() -> (w3464:string)
                n2673 = call <vilib>:"Write Characters To File.vi"("append to file? (new file:F)"=FALSE, "character string"=w3464, "file path (dialog if empty)"=w3469) -> ()  [unwired: 2 in, 1 out]
              }
            }
          }
          frame Enabled {
          }
        }
        n2674 = case shown="True" "OK Button 17" {
          frame False {
          }
          frame True {
            (unwired) 0  # existing file
            w3722 = "Choose a datalog file to open"  # prompt
            n2675 = local write "OK Button 17"(FALSE ("OK Button 17")) -> ()
            n2676 = local read "String"() -> (w3717:string)
            n2677 = String To Path(string=w3717) -> (path=w3718:path)
            n2678 = File Dialog(6:"*.duf" ("pattern"), 7:w3722, 11:w3718) -> (0:w3709:errorcluster, 3:w3728:path)  [unwired: 4 in, 2 out]
            n2679 = Unbundle(w3709) -> ()  [unwired: 3 out]
            n2680 = Open/Create/Replace File "Open File"(file path (use dialog)=w3728) -> (refnum out=w3720:refnum<file>)  [unwired: 5 in, 2 out]
            n2681 = Strip Path(path=w3728) -> (name=w3726:string)  [unwired: 1 out]
            n2682 = Path To String(path=w3728) -> (string=w3711:string)
            n2683 = while {
              tunnel: w3720 -> [w3732]
              i -> [w3729]
              stop <- w3730 continue-if-true
              (unwired) TRUE ("line mode (F)")
              n2684 = Read from Text File "Read File"(file (use dialog)=w3732) -> (text=w3731:string)  [unwired: 3 in, 3 out]
              n2685 = local write "Numeric 16"(w3729) -> ()
              n2686 = String Length(string=w3731) -> (length=w3734:i32)
              n2687 = Greater?(x=w3734, y=1) -> (0:w3730:bool)
            }
            n2688 = local write "String 29"(w3711) -> ()
            n2689 = Search and Replace String(input string=w3711, search string=".duf", replace string=".dgf" ("replace string (\"\")")) -> (result string=→"String Indicator 4":string)  [unwired: 5 in, 3 out]
            n2690 = Match Pattern(string=w3726, regular expression=".dwm") -> (before substring=w3710:string)  [unwired: 1 in, 3 out]
            "String Indicator" <- w3710
            n2691 = Match Pattern(string=w3711, regular expression=".dwm" ("substring (\"\")")) -> (before substring=w3712:string)  [unwired: 1 in, 3 out]
            "String Indicator 3" <- w3712
            n2692 = local write "TITTLE 2"(w3710) -> ()
            n2693 = String To Path(string=w3712) -> (path=w3719:path)
            "path" <- w3719
            n2694 = call <vilib>:"Read Characters From File.vi"("file path (dialog if empty)"=w3719, "start of read offset (chars.:0)"=60 ("start of read offset (chars.: 0)")) -> ("character string"=→"String Indicator 2":string)  [unwired: 4 in, 3 out]
          }
        }
        n2695 = call <vilib>:"Query Available Printers.vi"() -> ("system configured printers"=w3411:string[])  [unwired: 9 in, 2 out]
        "System Configured Printers 2" <- w3411
        n2696 = local read "OK Button 16"() -> (w3408:bool)
        n2697 = case shown="True" "OK Button 16" {
          frame False {
          }
          frame True {
            n2698 = stacked-sequence {
              frame #0 {
                n2699 = local read "Numeric 16"() -> (w3736:i32)
                n2700 = local write "Numeric 10"(w3736) -> ()
              }
              frame #1 {
                n2701 = local read "S.NO"() -> (→"s.NO":string)
                n2702 = local read "String 29"() -> (w3740:string)
                n2703 = String To Path(string=w3740) -> (path=w3739:path)
                n2704 = Open/Create/Replace File "Open File"(file path (use dialog)=w3739) -> (refnum out=w3741:refnum<file>)  [unwired: 5 in, 2 out]
                n2705 = for {
                  N: 16 -> [_]
                  tunnel: w3741 -> [w3748]
                  i -> [w3744]
                  (unwired) TRUE ("line mode (F)")
                  n2706 = Read from Text File "Read File"(file (use dialog)=w3748) -> (text=w3742:string)  [unwired: 3 in, 3 out]
                  n2707 = Match Pattern(string=w3742, regular expression="(") -> (after substring=w3747:string)  [unwired: 1 in, 3 out]
                  n2708 = Match Pattern(string=w3747, regular expression=")") -> (before substring=w3743:string)  [unwired: 1 in, 3 out]
                  n2709 = case shown="1" w3744 {
                    tunnel: w3743 -> [w3749 w3750 _ _ w3751 w3752 w3753 w3755 w3757 w3759 w3761 w3763 w3765 w3767 _]
                    tunnel: w3742 -> [_ _ _ _ _ _ _ _ _ _ _ _ _ _ _]
                    frame 0 {
                      "TITTLE" <- w3749
                    }
                    frame 1 {
                      "Sample ID" <- w3750
                    }
                    frame 2 {
                    }
                    frame 3 {
                    }
                    frame 4 {
                      "Test Date" <- w3751
                    }
                    frame 5 {
                      "Tested by" <- w3752
                    }
                    frame 6 {
                      n2710 = Fract/Exp String To Number(string=w3753) -> (number=→"Humidity before test 2":dbl)  [unwired: 3 in, 1 out]
                    }
                    frame 7 {
                      n2711 = Fract/Exp String To Number(string=w3755) -> (number=→"Temperature before test 2":dbl)  [unwired: 3 in, 1 out]
                    }
                    frame 8 {
                      n2712 = Fract/Exp String To Number(string=w3757) -> (number=→"Humidity after test 2":dbl)  [unwired: 3 in, 1 out]
                    }
                    frame 9 {
                      n2713 = Fract/Exp String To Number(string=w3759) -> (number=→"Temperature after test 2":dbl)  [unwired: 3 in, 1 out]
                    }
                    frame 10 {
                      n2714 = Fract/Exp String To Number(string=w3761) -> (number=→"MWSD 2":dbl)  [unwired: 3 in, 1 out]
                    }
                    frame 11 {
                      n2715 = Fract/Exp String To Number(string=w3763) -> (number=→"AVP 2":dbl)  [unwired: 3 in, 1 out]
                    }
                    frame 12 {
                      n2716 = Fract/Exp String To Number(string=w3765) -> (number=→"HCF 2":dbl)  [unwired: 3 in, 1 out]
                    }
                    frame 13 {
                      n2717 = Fract/Exp String To Number(string=w3767) -> (number=→"WS1.4 2":dbl)  [unwired: 3 in, 1 out]
                    }
                    frame 14, Default {
                    }
                  }
                }
              }
              frame #2 {
              }
            }
            n2718 = local write "OK Button 16"(FALSE ("OK Button 13")) -> ()
          }
        }
        n2719 = Index Array(array=w3411, index="Select Printer 3") -> (element=w3413:string)
